vi "AddTargetsConfigurationFile.vi"(8 "error in (no error)":errorcluster, 11 "VeriStandTestCase in":refnum<class "VeriStandTestCase.lvclass">) -> (0 "error out":errorcluster, 3 "VeriStandTestCase out":refnum<class "VeriStandTestCase.lvclass">)   [LabVIEW 2027, in "VeriStandTestCase.lvclass"]
uses:
  VeriStandTestCase.lvclass
  VeriStandTestCase.lvclass/VeriStandTestCase.ctl
  <userlib>/_OpenG.lib/file/file.llb/File Exists - Scalar__ogtk.vi
  VeriStandTestUtilities/VeriStandTestUtilities.lvlib
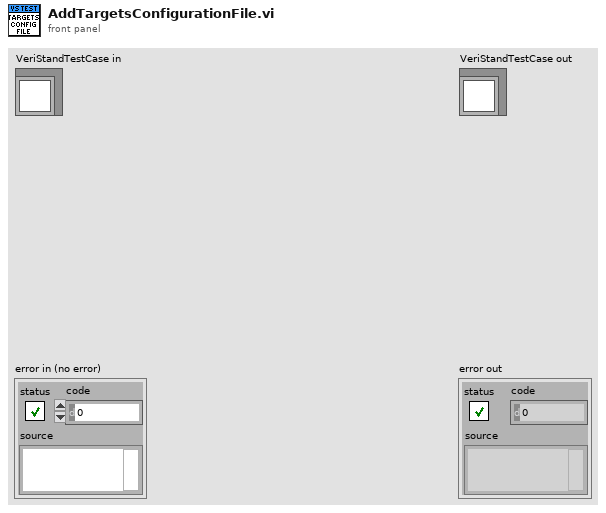
[diagram p1: front panel]
types:
  T1 = typedef "VeriStandTestUtilities.lvlib/TargetsConfiguration.ctl" = cluster{"Supported Targets":cluster{"IP Address / Hostname":string, "Target Platform":T2}[], "Active Configuration":T2}
  T2 = typedef "VeriStandTestUtilities.lvlib/TargetPlatform.ctl" = enum16{"Windows", "Linux64CRIO", "Linux64PXI", "LinuxARM", "PharLap"}
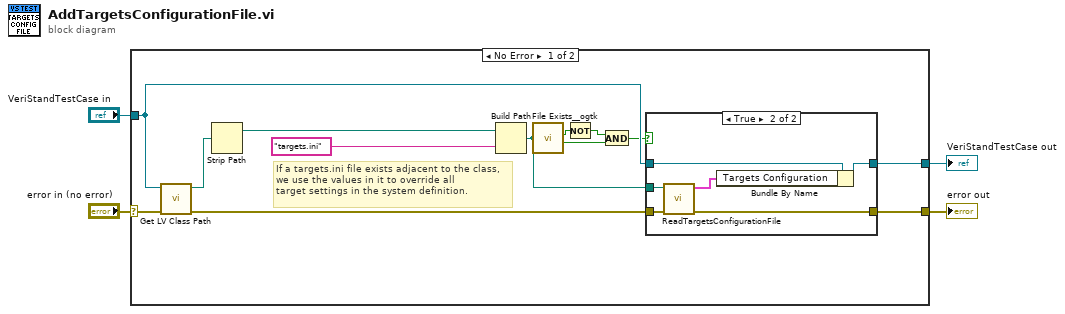
[diagram p0: block diagram]
diagram:
  n1 = case shown="No Error" "error in (no error)" {
    selector: "error in (no error)" -> [w14 w27]
    tunnel: [w16 w27] -> w3
    tunnel: [w17 w26] -> w1
    tunnel: "VeriStandTestCase in" -> [w15 w26]
    frame No Error {
      # "If a targets.ini file exists adjacent to the class,\nwe use the values in it to override all\ntarget settings in the system definition."
      n2 = call <vilib>:"Get LV Class Path.vi"("error in (no error)"=w14, "object"=w15) -> ("error out"=w13:errorcluster, "class path"=w12:path)  [unwired: 8 in]
      n3 = Strip Path(path=w12) -> (stripped path=w10:path)  [unwired: 1 out]
      n4 = Build Path(base path=w10, name or relative path="targets.ini") -> (appended path=w5:path)
      n5 = call-poly <userlib>:"File Exists__ogtk.vi"("file path"=w5) -> ("is directory"=w9:bool, "exists"=w7:bool)  [unwired: 6 in]
      n6 = Not(x=w9) -> (.not. x?=w8:bool)
      n7 = And(x=w8, y=w7) -> (x .and. y?=w6:bool)
      n8 = case shown="True" w6 {
        tunnel: w15 -> [w18 w25]
        tunnel: [w18 w24] -> w17
        tunnel: w13 -> [w19 w22]
        tunnel: [w19 w23] -> w16
        tunnel: w5 -> [_ w21]
        frame False {
        }
        frame True {
          n9 = call "ReadTargetsConfigurationFile.vi"("error in (no error)"=w22, "targets.ini file"=w21) -> ("error out"=w23:errorcluster, "Targets Configuration"=w20:T1)  [unwired: 8 in]
          n10 = Bundle By Name(cluster=w25, "Targets Configuration"=w20) -> (w24:refnum<class "VeriStandTestCase.lvclass">)
        }
      }
    }
    frame Error {
    }
  }
  "error out" <- w3
  "VeriStandTestCase out" <- w1
